vi "TP_FINAL_control_manual.vi"() -> ()   [LabVIEW 2025]
uses:
  <vilib>/Instr/_visa.llb/VISA Configure Serial Port (Instr).vi
panel:
  out "Intensidad":dbl(ramp)
  out "Brillo":dbl format="%#_4g"
  out "Gráfica de brillo":dbl(graph)
  in  "Knob":dbl(knob) min=0.0 max=255.0 scale=0.0..100.0
  in  "stop":bool
  in  "VISA resource name":refnum<visa-resource-name>
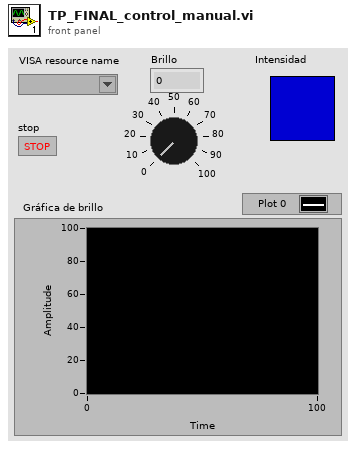
[diagram p1: front panel]
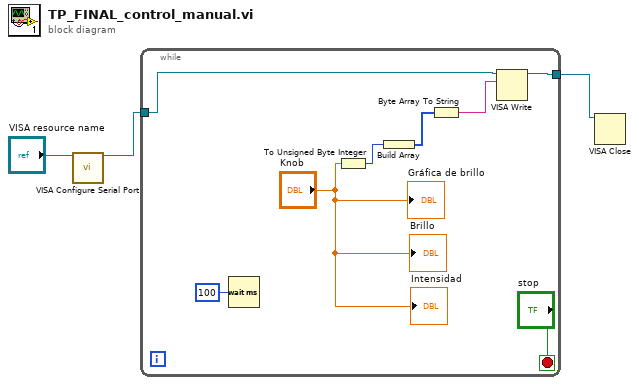
[diagram p0: block diagram]
diagram:
  n1 = call-poly "VISA Configure Serial Port"("VISA resource name"="VISA resource name") -> ("VISA resource name out"=w2:refnum<visa-resource-name>)  [unwired: 13 in, 1 out]
  n2 = while {
    tunnel: w2 -> [w11]
    tunnel: [w9] -> w1
    stop <- "stop" stop-if-true
    n3 = Wait (ms)(milliseconds to wait=u32 100) -> ()  [unwired: 1 out]
    n4 = To Unsigned Byte Integer(number="Knob") -> (unsigned 8bit integer=w6:u8)
    n5 = Build Array(w6) -> (w7:u8[])
    n6 = Byte Array To String(unsigned byte array=w7) -> (string=w4:string)
    n7 = VISA Write(VISA resource name=w11, write buffer=w4) -> (VISA resource name out=w9:refnum<visa-resource-name>)  [unwired: 1 in, 2 out]
    "Gráfica de brillo" <- "Knob"
    "Brillo" <- "Knob"
    "Intensidad" <- "Knob"
  }
  n8 = VISA Close(VISA resource name=w1) -> ()  [unwired: 1 in, 1 out]
